vi "Pack Frame Data.vi"(8 "Error In":errorcluster, 11 "Data Frame":T1) -> (0 "Error Out":errorcluster, 3 "Packed Data":u64)   [LabVIEW 2021, in "Display.lvclass"]
uses:
  Display.lvclass
  Display.lvclass/Display.ctl
  Shared/Public/Controls/Neopixel FIFO Command.ctl
  Shared/Neopixel Shared.lvlib
  Shared/Public/Controls/Data Frame.ctl
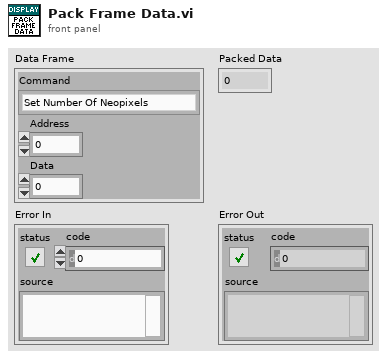
[diagram p1: front panel]
types:
  T1 = typedef "Neopixel Shared.lvlib/Data Frame.ctl" = cluster{"Command":T2, "Address":u16, "Data":u32}
  T2 = typedef "Neopixel Shared.lvlib/Neopixel FIFO Command.ctl" = enum8{"Set Number Of Neopixels", "Update Frame"}
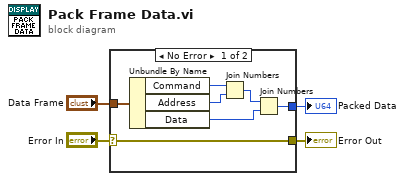
[diagram p0: block diagram]
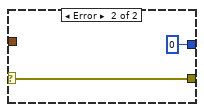
[diagram p2: hidden frame]
diagram:
  n1 = case shown="No Error" "Error In" {
    selector: "Error In" -> [w5 w13]
    tunnel: [w11 u64 0] -> w4
    tunnel: "Data Frame" -> [w6 _]
    tunnel: [w5 w13] -> w1
    frame No Error {
      n2 = Unbundle By Name(w6) -> ("Command"=w7:T2, "Address"=w8:u16, "Data"=w9:u32)
      n3 = Join Numbers(hi=w7, lo=w8) -> ((hi.lo)=w10:u32)
      n4 = Join Numbers(hi=w10, lo=w9) -> ((hi.lo)=w11:u64)
    }
    frame Error {
    }
  }
  "Packed Data" <- w4
  "Error Out" <- w1
